vi "Initialize.vi"(2 "error in (no error)":errorcluster, 4 "Reset (True)":bool=TRUE, 5 "KE_In":refnum<visa-resource-name>) -> (0 "error out":errorcluster, 1 "KE_Out":refnum<visa-resource-name>)   [LabVIEW 2012]
uses:
  <instrlib>/Keithley 24XX/Keithley 24XX.lvlib
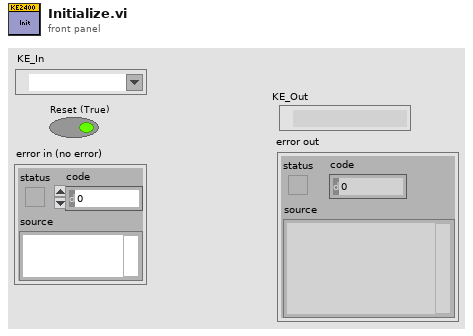
[diagram p1: front panel]
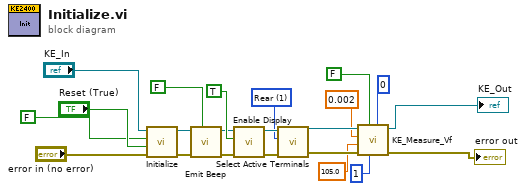
[diagram p0: block diagram]
diagram:
  w13 = u16 1 items=["Front", "Rear"] ("Active Terminals (0: Front)")
  n1 = call <instrlib>:"Initialize.vi"("error in (no error)"="error in (no error)", "Reset (True)"="Reset (True)", "ID Query (True)"=FALSE, "VISA resource name"="KE_In") -> ("error out"=w18:errorcluster, "VISA resource name out"=w19:refnum<visa-resource-name>)  [unwired: 6 in]
  n2 = call <instrlib>:"Emit Beep.vi"("Enable Beep (F)"=FALSE, "error in (no error)"=w18, "VISA resource name"=w19) -> ("error out"=w15:errorcluster, "VISA resource name out"=w16:refnum<visa-resource-name>)  [unwired: 7 in]
  n3 = call <instrlib>:"Enable Display.vi"("error in (no error)"=w15, "Enable Display (T: Enable)"=TRUE, "VISA resource name"=w16) -> ("error out"=w12:errorcluster, "VISA resource name out"=w14:refnum<visa-resource-name>)  [unwired: 7 in]
  n4 = call <instrlib>:"Select Active Terminals.vi"("error in (no error)"=w12, "Active Terminals (0: Front)"=w13, "VISA resource name"=w14) -> ("error out"=w9:errorcluster, "VISA resource name out"=w10:refnum<visa-resource-name>)  [unwired: 7 in]
  n5 = call "KE_Measure_Vf.vi"("Settle Delay"=u32 0, "Samples"=1, "Keep On"=FALSE, "error in (no error)"=w9, "Compliance"=105.0, "Current(A)"=0.002, "KE_In"=w10) -> ("error out"=→"error out":errorcluster, "KE_Out"=→"KE_Out":refnum<visa-resource-name>)  [unwired: 2 in, 1 out]
